vi "Event Queue Self Alias.vi"(11 "Base Event jettl in":refnum<class "Base Event jettl.lvclass">) -> (2 "Queue Self Alias":string, 3 "Base Event jettl out":refnum<class "Base Event jettl.lvclass">)   [LabVIEW 2021, in "jettl.lvlib" / "Base Event jettl.lvlib" / "Base Event jettl.lvclass"]
uses:
  Base Event jettl.lvclass
  Base Event jettl.lvclass/Base Event jettl.ctl
  jettl.lvlib
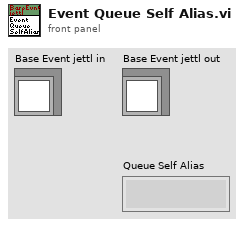
[diagram p1: front panel]
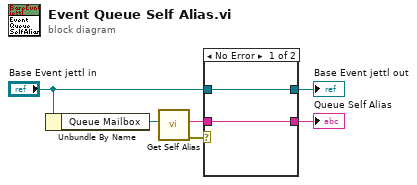
[diagram p0: block diagram]
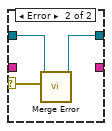
[diagram p2: hidden frame]
diagram:
  n1 = Unbundle By Name("Base Event jettl in") -> ("Queue Mailbox"=w4:refnum<data-value>)
  n2 = call "Get Self Alias.vi"("Queue Mailbox"=w4) -> ("error out"=w6:errorcluster, "Self Alias"=w5:string)  [unwired: 9 in]
  n3 = case shown="No Error" w6 {
    selector: w6 -> [_ w9]
    tunnel: [w8 w10] -> w2
    tunnel: "Base Event jettl in" -> [w8 w11]
    tunnel: [w7 _] -> w1
    tunnel: w5 -> [w7 _]
    frame No Error {
    }
    frame Error {
      n4 = call-dynamic "Merge Error.vi"("Error"=w9, "Base Event jettl in"=w11) -> ("Base Event jettl out"=w10:refnum<class "Base Event jettl.lvclass">)  [unwired: 9 in]
    }
  }
  "Base Event jettl out" <- w2
  "Queue Self Alias" <- w1
